vi "Read indent.vi"(11 "MsgSerializer in":refnum<class "MsgSerializer.lvclass">) -> (2 "indent":i32, 3 "MsgSerializer out":refnum<class "MsgSerializer.lvclass">)   [LabVIEW 2013, in "Caraya.lvlib" / "MsgSerializer.lvclass"]
uses:
  MsgSerializer.lvclass
  MsgSerializer.lvclass/MsgSerializer.ctl
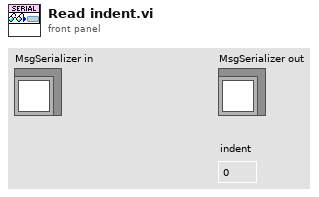
[diagram p1: front panel]
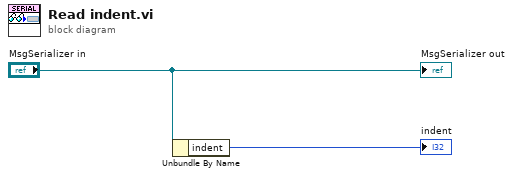
[diagram p0: block diagram]
diagram:
  n1 = Unbundle By Name("MsgSerializer in") -> ("indent"=→"indent":i32)
  "MsgSerializer out" <- "MsgSerializer in"
